vi "GraphWindow_LS1.vi"() -> (11 "Graph":cluster{dbl[], dbl[]}[](graph))   [LabVIEW 2019]
uses:
  Interface Class/PlotChange.ctl
panel:
  in  "MainGraphQ":refnum<queue>
  in  "Graph Event":refnum<user-event>
  in  "GraphQRef":refnum<queue>
  out "error out":errorcluster caption="sortie d'erreur"
  in  "error in (no error)":errorcluster
  in  "stop":bool
  in  "ToolsVis":bool
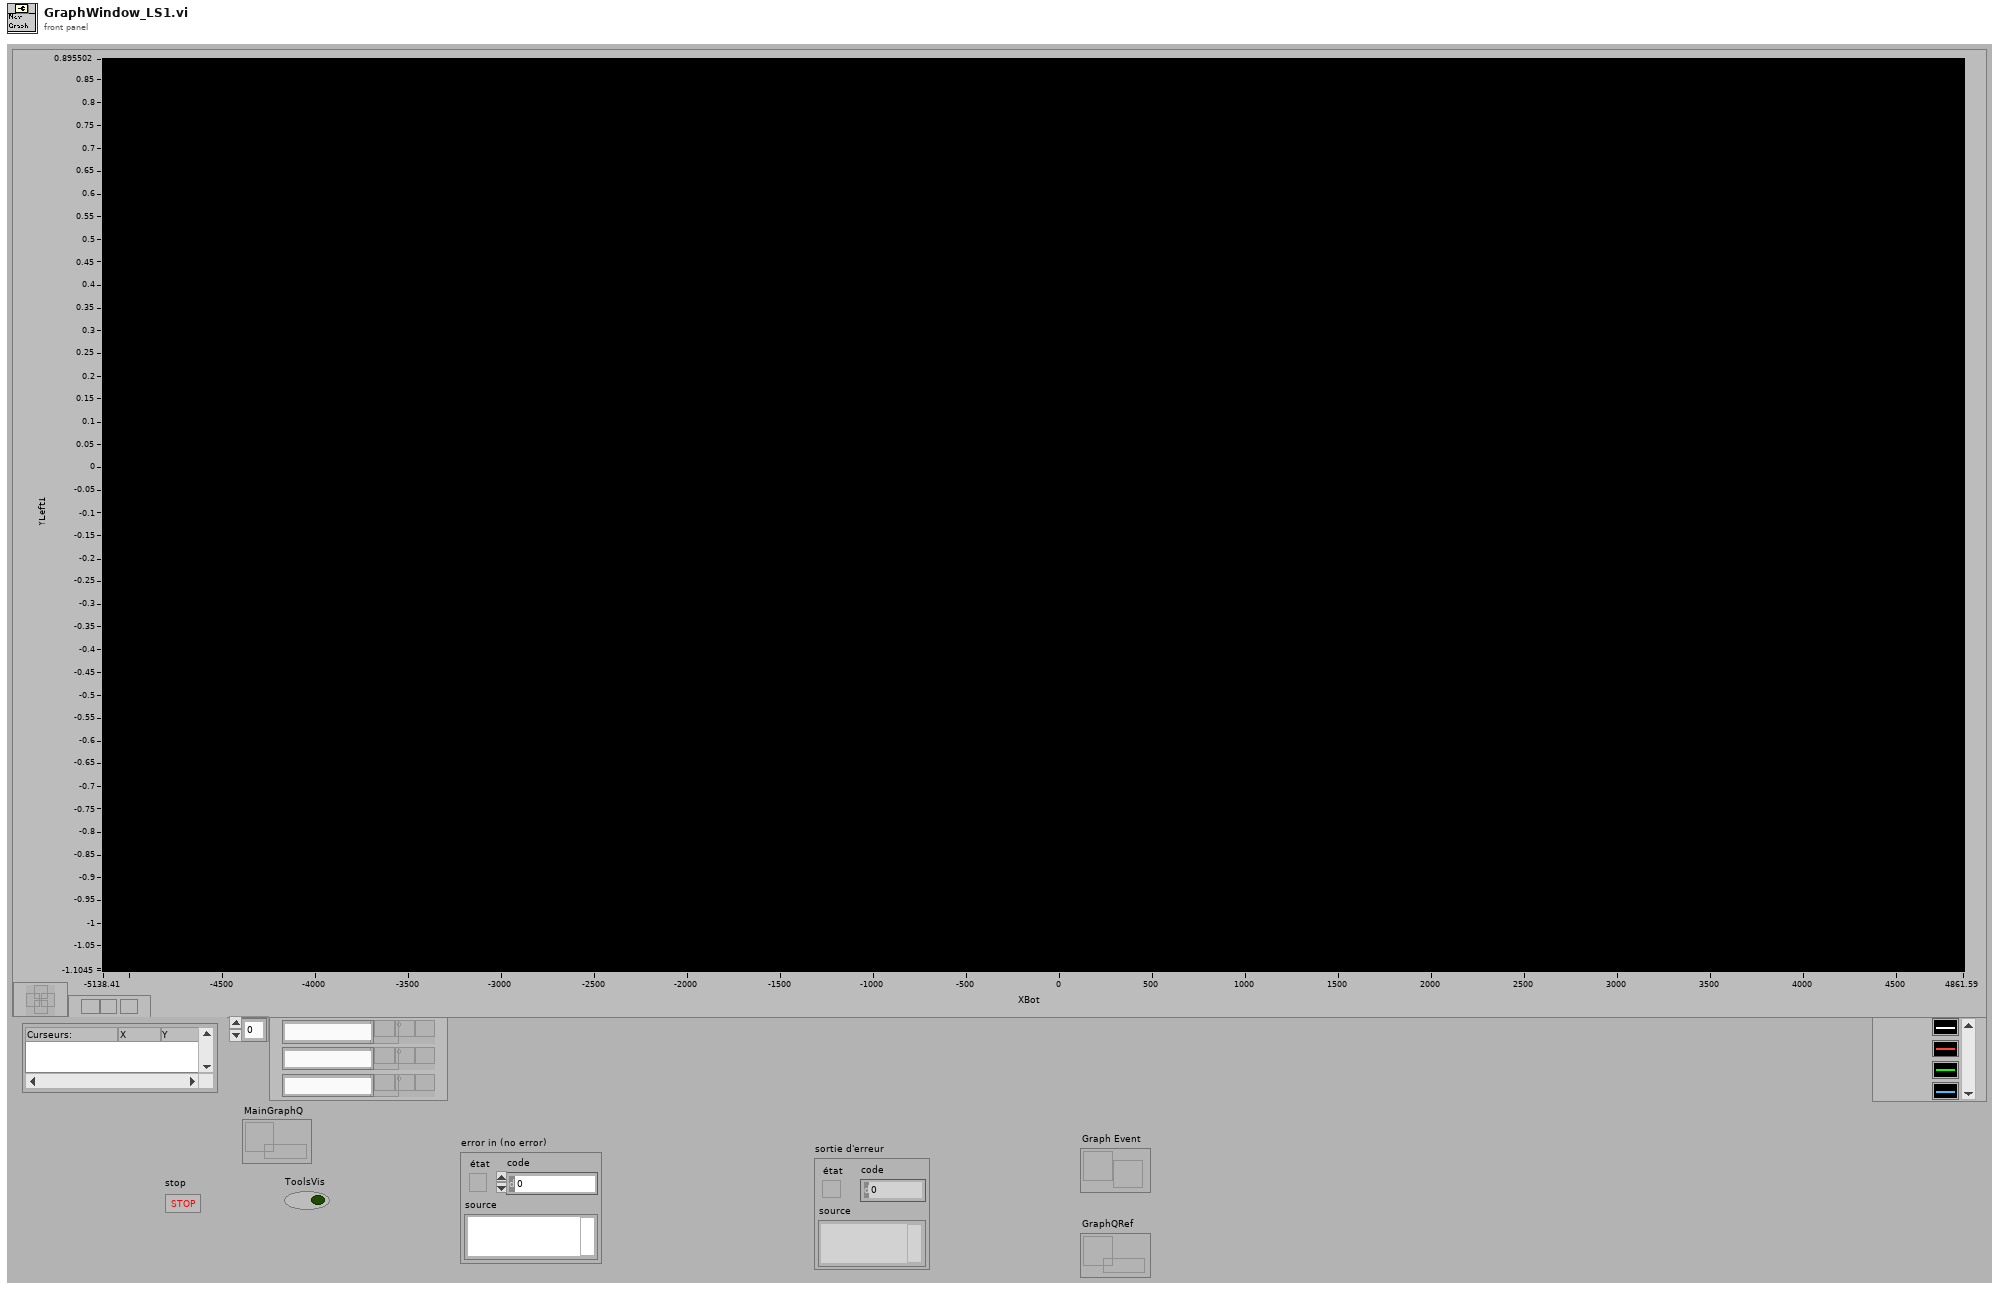
[diagram p1: front panel]
types:
  T1 = cluster{"Message":string, "Data":variant, i32, cluster{dbl[], dbl[]}[]}
  T2 = typedef "PlotChange.ctl" = cluster{"PlotIdx":i32, "PlotAttrib":cluster{"Color":u32, "PointStyle":u8, "LineStyle":u8, "Interp":u8, "LineWidth":u8, "BarPlotStyle":u8, "FillTo":i16, "XScaleIdx":u32, "YScaleIdx":u32, "Anti-Aliased":bool, "LabelFormat":u8, "TransitionType":u8, "TransitionLocation":u8, "DigitalLineStyle":u8}, "GraphId":i32, "Crv Visible":bool}
  T3 = cluster{"Color":u32, "PointStyle":u8, "LineStyle":u8, "Interp":u8, "LineWidth":u8, "BarPlotStyle":u8, "FillTo":i16, "XScaleIdx":u32, "YScaleIdx":u32, "Anti-Aliased":bool, "LabelFormat":u8, "TransitionType":u8, "TransitionLocation":u8, "DigitalLineStyle":u8}
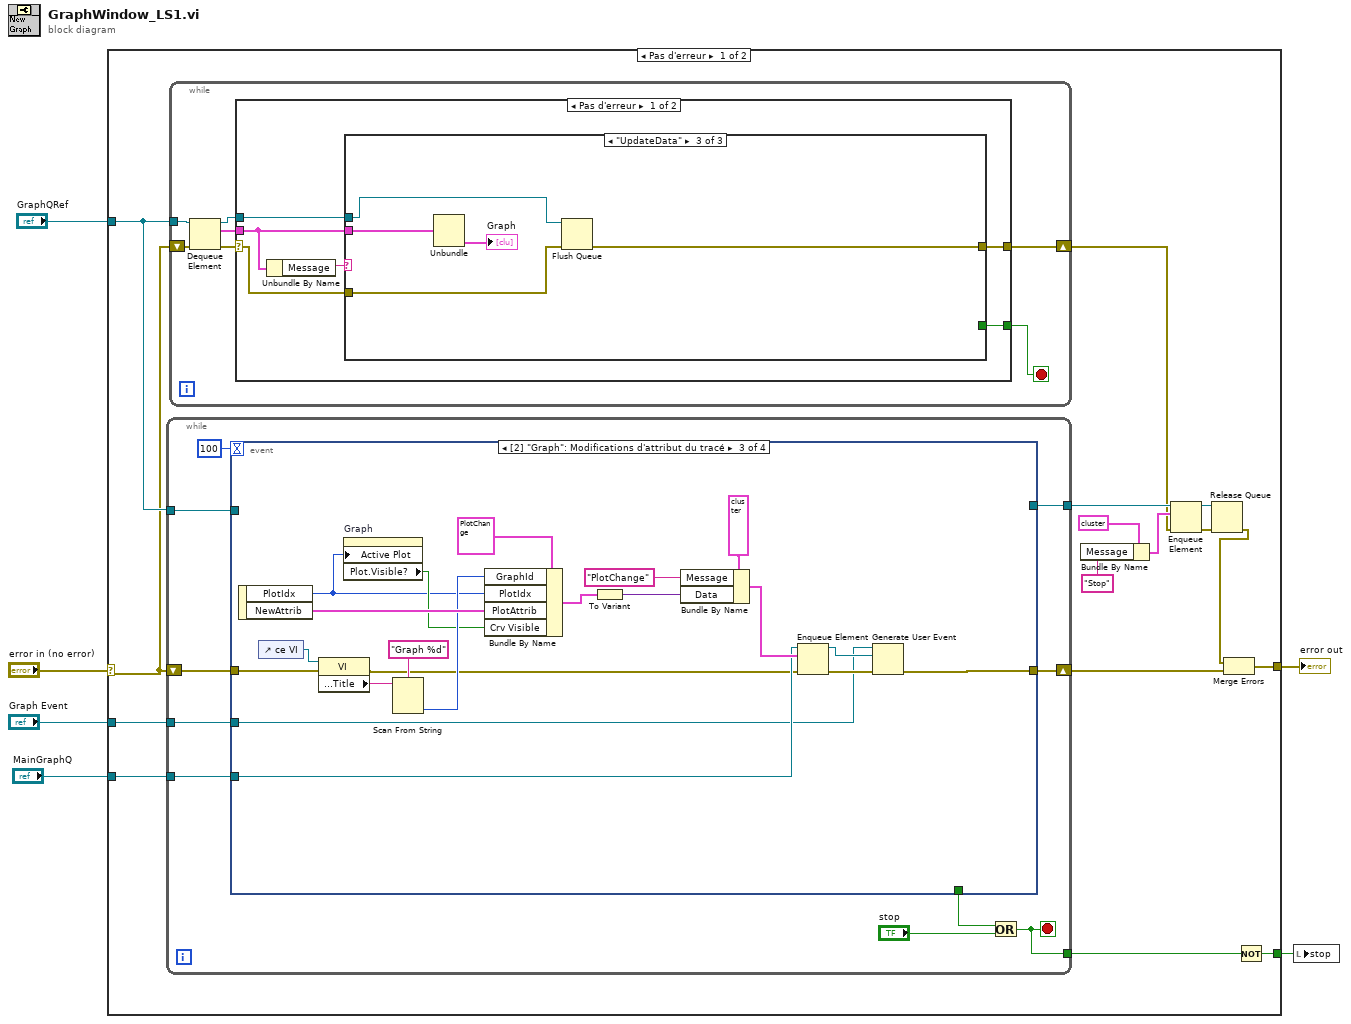
[diagram p0: block diagram]
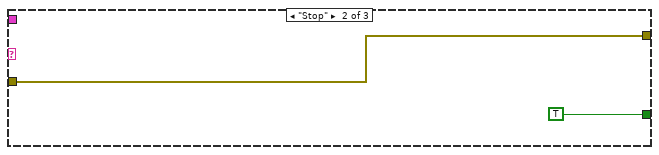
[diagram p3: hidden frame]
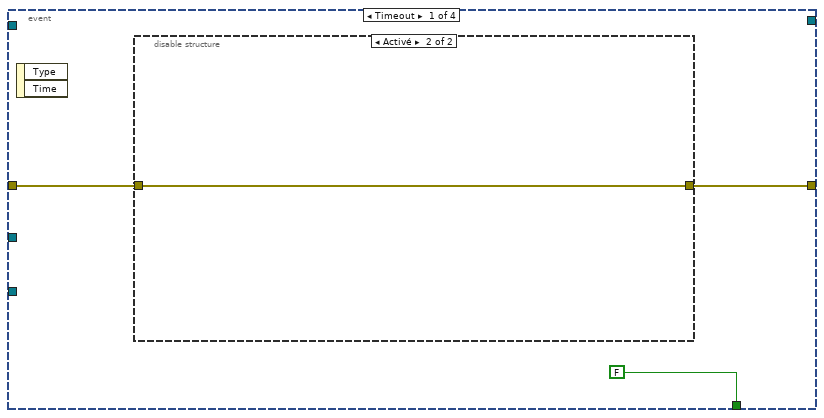
[diagram p5: hidden frame]
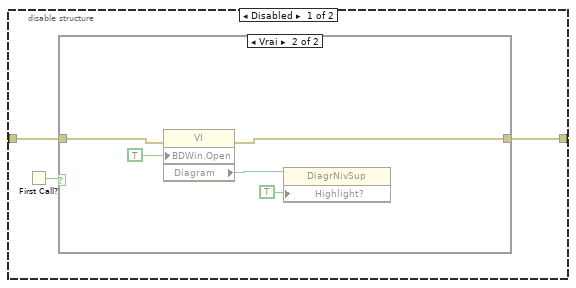
[diagram p6: hidden frame]
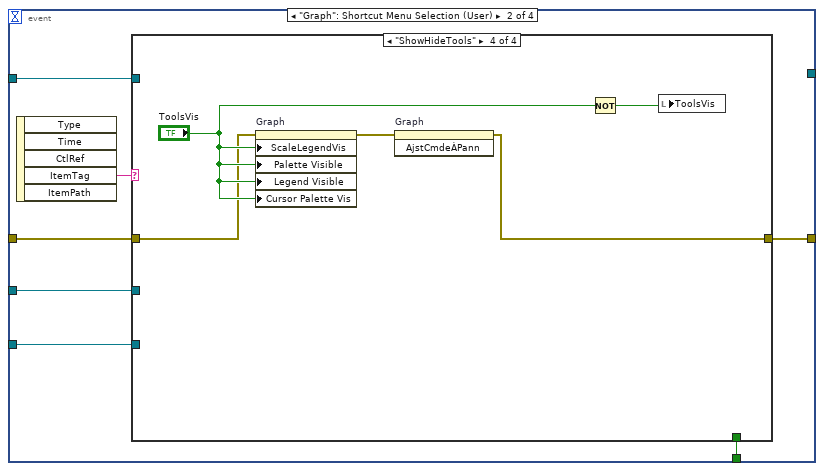
[diagram p8: hidden frame]
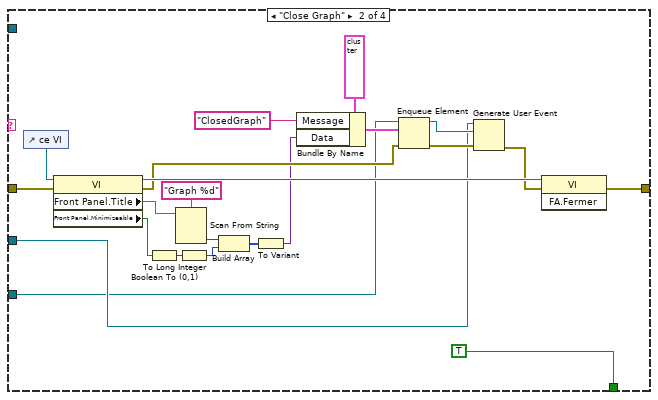
[diagram p10: hidden frame]
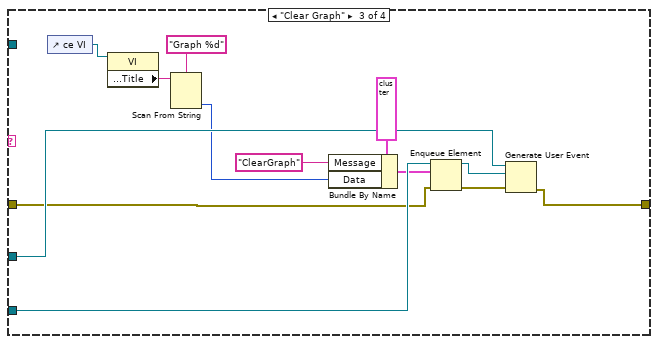
[diagram p11: hidden frame]
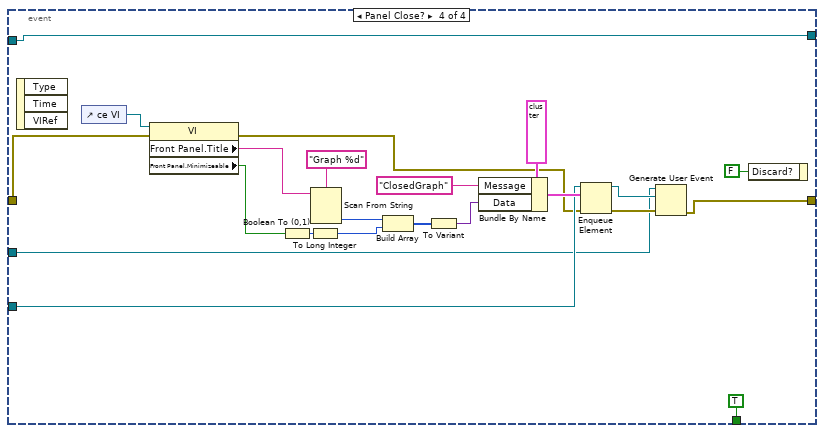
[diagram p12: hidden frame]
diagram:
  n1 = case shown="Pas d'erreur" "error in (no error)" {
    selector: "error in (no error)" -> [w9 w158]
    tunnel: [w14 w158] -> w5
    tunnel: [w21 _] -> w4
    tunnel: "GraphQRef" -> [w19 _]
    tunnel: "Graph Event" -> [w8 _]
    tunnel: "MainGraphQ" -> [w7 _]
    frame No Error {
      n2 = while {
        shift-right: [w51] -> w20
        shift-left: w9 -> [w52]
        tunnel: [w50] -> w22
        tunnel: w19 -> [w49]
        tunnel: [w48] -> w18
        tunnel: w8 -> [w47]
        tunnel: w7 -> [w46]
        stop <- w50 stop-if-true
        n3 = event shown="[2] \"Graph\": Modifications d'attribut du tracé" {
          selector: _ -> [_ _ _ _]
          dyn-events: _ -> [_ _ _ _]
          timeout: 100 -> [_ _ _ _]
          tunnel: [FALSE w73 _ TRUE] -> w54
          tunnel: w52 -> [w56 w72 w130 w154]
          tunnel: [w55 w71 w119 w142] -> w51
          tunnel: w49 -> [_ w70 _ w151]
          tunnel: [_ _ _ w151] -> w48
          tunnel: w47 -> [_ w69 w120 w143]
          tunnel: w46 -> [_ w68 w121 w144]
          event Timeout {
            n4 = event-data() -> ()  [unwired: 1 in, 2 out]
            n5 = disable-structure shown="Activé" {
              disable-tunnel: w56 -> [w60 w67]
              disable-tunnel: [w59 w67] -> w55
              frame Disabled {
                n6 = First Call?() -> (First Call?: T/F=w58:bool)
                n7 = case shown="Vrai" w58 {
                  tunnel: w60 -> [w61 w65]
                  tunnel: [w61 w64] -> w59
                  frame False {
                  }
                  frame True {
                    n8 = property class="VI"(error in=w65, "BDWin.Open"=TRUE ("Fenêtre du diagramme : ouverte")) -> (error out=w64:errorcluster, "Diagram"=w63:refnum<vi>)  [unwired: 1 in, 1 out]
                    n9 = property class="DiagrNivSup"(reference=w63, "Highlight?"=TRUE ("Animer l'exécution ?")) -> ()  [unwired: 1 in, 2 out]
                  }
                }
              }
              frame Enabled {
              }
            }
          }
          event "Graph": Shortcut Menu Selection (User) {
            n10 = event-data() -> ("ItemTag"=w74:string)  [unwired: 1 in, 4 out]
            n11 = case shown="\"ShowHideTools\"" w74 {
              tunnel: [_ TRUE _ _] -> w73
              tunnel: w72 -> [w75 w93 w106 w112]
              tunnel: [w75 w92 w105 w111] -> w71
              tunnel: w70 -> [_ _ _ _]
              tunnel: w69 -> [_ w82 w108 _]
              tunnel: w68 -> [_ w81 w107 _]
              frame Default {
              }
              frame "Close Graph" {
                n12 = control-ref of="ce VI"() -> (w79:refnum<vi>)
                n13 = property class="VI"(reference=w79, error in=w93) -> (reference out=w94:refnum<vi>, error out=w84:errorcluster, "Front Panel.Title"=w95:string, "Front Panel.Minimizeable"=w78:bool)
                n14 = Boolean To (0,1)(Boolean=w78) -> (0, 1=w77:i16)
                n15 = Scan From String(format string="Graph %d" ("chaîne de format"), input string=w95) -> (output 1=w91:i32)  [unwired: 3 in, 3 out]
                n16 = To Long Integer(number=w77) -> (32bit integer=w76:i32)
                n17 = Build Array(w91, w76) -> (w80:i32[])
                n18 = To Variant(anything=w80) -> (Variant=w83:variant)
                n19 = Bundle By Name(cluster=cluster{"Message":string, "Data":variant, i32} {"Message"="", "Data"=variant, 0} ("ClassQueue"), "Message"="ClosedGraph", "Data"=w83) -> (w87:cluster{"Message":string, "Data":variant, i32})
                n20 = Enqueue Element(queue=w81, element=w87, error in (no error)=w84) -> (queue out=w89:refnum<queue>, error out=w90:errorcluster)  [unwired: 1 in, 1 out]
                n21 = Generate User Event(user event=w82, event data cluster=w89, error in=w90) -> (error out=w85:errorcluster)  [unwired: 1 in, 1 out]
                n22 = invoke class="VI" method="FA.Fermer"(reference=w94, error in=w85) -> (error out=w92:errorcluster)  [unwired: 1 in, 2 out]
              }
              frame "Clear Graph" {
                n23 = control-ref of="ce VI"() -> (w100:refnum<vi>)
                n24 = property class="VI"(reference=w100) -> ("Front Panel.Title"=w101:string)  [unwired: 1 in, 2 out]
                n25 = Scan From String(format string="Graph %d" ("chaîne de format"), input string=w101) -> (output 1=w99:i32)  [unwired: 3 in, 3 out]
                n26 = Bundle By Name(cluster=cluster{"Message":string, "Data":variant, i32} {"Message"="", "Data"=variant, 0} ("ClassQueue"), "Message"="ClearGraph", "Data"=w99) -> (w103:cluster{"Message":string, "Data":variant, i32})
                n27 = Enqueue Element(queue=w107, element=w103, error in (no error)=w106) -> (queue out=w109:refnum<queue>, error out=w110:errorcluster)  [unwired: 1 in, 1 out]
                n28 = Generate User Event(user event=w108, event data cluster=w109, error in=w110) -> (error out=w105:errorcluster)  [unwired: 1 in, 1 out]
              }
              frame "ShowHideTools" {
                n29 = property on="Graph" class="GraphXY (strict)"(error in=w112, "ScaleLegendVis"="ToolsVis", "Palette Visible"="ToolsVis", "Legend Visible"="ToolsVis", "Cursor Palette Vis"="ToolsVis") -> (error out=w113:errorcluster)  [unwired: 1 in, 1 out]
                n30 = invoke on="Graph" class="GraphXY (strict)" method="AjstCmdeÀPann"(error in=w113) -> (error out=w111:errorcluster)  [unwired: 2 in, 2 out]
                n31 = Not(x="ToolsVis") -> (.not. x?=w115:bool)
                n32 = local write "ToolsVis"(w115) -> ()
              }
            }
          }
          event "Graph": Plot Attribute Change {
            n33 = event-data() -> ("PlotIdx"=w116:i32, "NewAttrib"=w134:T3)  [unwired: 1 in]
            n34 = control-ref of="ce VI"() -> (w131:refnum<vi>)
            n35 = property class="VI"(reference=w131, error in=w130) -> (error out=w118:errorcluster, "Front Panel.Title"=w132:string)  [unwired: 1 out]
            n36 = property on="Graph" class="GraphXY (strict)"("Active Plot"=w116) -> ("Plot.Visible?"=w117:bool)  [unwired: 2 in, 2 out]
            n37 = Scan From String(format string="Graph %d" ("chaîne de format"), input string=w132) -> (output 1=w129:i32)  [unwired: 3 in, 3 out]
            n38 = Bundle By Name(cluster=T2 {"PlotIdx"=0, "PlotAttrib"={"Color"=0, "PointStyle"=0, "LineStyle"=0, "Interp"=0, "LineWidth"=0, "BarPlotStyle"=0, "FillTo"=0, "XScaleIdx"=0, "YScaleIdx"=0, "Anti-Aliased"=FALSE, "LabelFormat"=0, "TransitionType"=0, "TransitionLocation"=0, "DigitalLineStyle"=0}, "GraphId"=0, "Crv Visible"=FALSE} ("Valeur"), "GraphId"=w129, "PlotIdx"=w116, "PlotAttrib"=w134, "Crv Visible"=w117) -> (w128:T2)
            n39 = To Variant(anything=w128) -> (Variant=w122:variant)
            n40 = Bundle By Name(cluster=cluster{"Message":string, "Data":variant, i32} {"Message"="", "Data"=variant, 0} ("ClassQueue"), "Message"="PlotChange", "Data"=w122) -> (w124:cluster{"Message":string, "Data":variant, i32})
            n41 = Enqueue Element(queue=w121, element=w124, error in (no error)=w118) -> (queue out=w126:refnum<queue>, error out=w127:errorcluster)  [unwired: 1 in, 1 out]
            n42 = Generate User Event(user event=w120, event data cluster=w126, error in=w127) -> (error out=w119:errorcluster)  [unwired: 1 in, 1 out]
          }
          event Panel Close? {
            n43 = event-data() -> ()  [unwired: 1 in, 3 out]
            n44 = control-ref of="ce VI"() -> (w139:refnum<vi>)
            n45 = property class="VI"(reference=w139, error in=w154) -> (error out=w141:errorcluster, "Front Panel.Title"=w156:string, "Front Panel.Minimizeable"=w136:bool)  [unwired: 1 out]
            n46 = Boolean To (0,1)(Boolean=w136) -> (0, 1=w138:i16)
            n47 = To Long Integer(number=w138) -> (32bit integer=w137:i32)
            n48 = Scan From String(format string="Graph %d" ("chaîne de format"), input string=w156) -> (output 1=w155:i32)  [unwired: 3 in, 3 out]
            n49 = Build Array(w155, w137) -> (w140:i32[])
            n50 = To Variant(anything=w140) -> (Variant=w145:variant)
            n51 = Bundle By Name(cluster=cluster{"Message":string, "Data":variant, i32} {"Message"="", "Data"=variant, 0} ("ClassQueue"), "Message"="ClosedGraph", "Data"=w145) -> (w147:cluster{"Message":string, "Data":variant, i32})
            n52 = Enqueue Element(queue=w144, element=w147, error in (no error)=w141) -> (queue out=w149:refnum<queue>, error out=w150:errorcluster)  [unwired: 1 in, 1 out]
            n53 = Generate User Event(user event=w143, event data cluster=w149, error in=w150) -> (error out=w142:errorcluster)  [unwired: 1 in, 1 out]
            n54 = event-data("Discard?"=FALSE ("Rejeter ?")) -> ()  [unwired: 1 in, 1 out]
          }
        }
        n55 = Or(x=w54, y="stop") -> (x .or. y?=w50:bool)
      }
      n56 = while {
        tunnel: w19 -> [w29]
        shift-right: [w26] -> w13
        shift-left: w9 -> [w27]
        stop <- w24 stop-if-true
        n57 = Dequeue Element(queue=w29, error in (no error)=w27) -> (queue out=w23:refnum<queue>, element=w25:T1, error out=w28:errorcluster)  [unwired: 1 in, 1 out]
        n58 = case shown="Pas d'erreur" w28 {
          selector: w28 -> [w35 w44]
          tunnel: [w31 w44] -> w26
          tunnel: w25 -> [w34 _]
          tunnel: [w32 _] -> w24
          tunnel: w23 -> [w30 _]
          frame No Error {
            n59 = Unbundle By Name(w34) -> ("Message"=w33:string)
            n60 = case shown="\"UpdateData\"" w33 {
              tunnel: w34 -> [_ _ w43]
              tunnel: [w36 w38 w40] -> w31
              tunnel: w35 -> [w36 w38 w41]
              tunnel: [_ TRUE _] -> w32
              tunnel: w30 -> [_ _ w39]
              frame Default {
              }
              frame "Stop" {
              }
              frame "UpdateData" {
                n61 = Unbundle(w43) -> (→"Graph":cluster{dbl[], dbl[]}[])  [unwired: 3 out]
                n62 = Flush Queue(queue=w39, error in (no error)=w41) -> (error out=w40:errorcluster)  [unwired: 2 out]
              }
            }
          }
          frame Error {
            # "timeout"
          }
        }
      }
      n63 = Bundle By Name(cluster=T1 {"Message"="", "Data"=variant, 0, []} ("élément"), "Message"="Stop") -> (w16:T1)
      n64 = Enqueue Element(queue=w18, element=w16, error in (no error)=w13) -> (queue out=w12:refnum<queue>, error out=w11:errorcluster)  [unwired: 1 in, 1 out]
      n65 = Release Queue(queue=w12, error in (no error)=w11) -> (error out=w10:errorcluster)  [unwired: 1 in, 2 out]
      n66 = Merge Errors(w10, w20) -> (w14:errorcluster)
      n67 = Not(x=w22) -> (.not. x?=w21:bool)
    }
    frame Error {
    }
  }
  "error out" <- w5
  n68 = local write "stop"(w4) -> ()
